vi "Delete Ansiotropic Filter 32f.vi"(8 "Error In":errorcluster, 11 "Anisotropic Filter Object":T1={"Device In"=0, "Convolution Object"={"Device In"=0, "Program Handle"=0, "Kernel Memory Object"={"Device ID"=0, "Memeroy ID"=0, "Dimension"={"Depth"=0, "Height"=0, "Width"=0}, "Memory Type"=enum."32f"}, "Convolved Memory Object"={"Device ID"=0, "Memeroy ID"=0, "Dimension"={"Depth"=0, "Height"=0, "Width"=0}, "Memory Type"=enum."32f"}}, "Imag Kernel"=[], "Real Kernel"=[], "Convolved Buffer"={"Device ID"=0, "Memeroy ID"=0, "Dimension"={"Depth"=0, "Height"=0, "Width"=0}, "Memory Type"=enum."32f"}, "Program Handle"=0, "Ansiotropic Filter Parameters"={"Time Step"=0.0, "Total Time"=0.5, "Std. Deviation"=0.0, "Gaussian Filter X Size"=1, "Gaussian Filter Y Size"=1, "Gaussian Filter Z Size"=1}, "Raw Data"={"Device ID"=0, "Memeroy ID"=0, "Dimension"={"Depth"=0, "Height"=0, "Width"=0}, "Memory Type"=enum."32f"}, "Buffer 3"={"Device ID"=0, "Memeroy ID"=0, "Dimension"={"Depth"=0, "Height"=0, "Width"=0}, "Memory Type"=enum."32f"}, "Dimensions"={"Depth"=1, "Height"=1, "Width"=1}} {"Dimensions"."Width" min=1; "Dimensions"."Height" min=1; "Dimensions"."Depth" min=1; "Buffer 3"."Dimension"."Width" min=1; "Buffer 3"."Dimension"."Height" min=1; "Buffer 3"."Dimension"."Depth" min=1; "Raw Data"."Dimension"."Width" min=1; "Raw Data"."Dimension"."Height" min=1; "Raw Data"."Dimension"."Depth" min=1; "Ansiotropic Filter Parameters"."Gaussian Filter Z Size" min=1 max=99 step=2; "Ansiotropic Filter Parameters"."Gaussian Filter Y Size" min=1 max=99 step=2; "Ansiotropic Filter Parameters"."Gaussian Filter X Size" min=1 max=99 step=2; "Convolved Buffer"."Dimension"."Width" min=1; "Convolved Buffer"."Dimension"."Height" min=1; "Convolved Buffer"."Dimension"."Depth" min=1; "Convolution Object"."Convolved Memory Object"."Dimension"."Width" min=1; "Convolution Object"."Convolved Memory Object"."Dimension"."Height" min=1; "Convolution Object"."Convolved Memory Object"."Dimension"."Depth" min=1; "Convolution Object"."Kernel Memory Object"."Dimension"."Width" min=1; "Convolution Object"."Kernel Memory Object"."Dimension"."Height" min=1; "Convolution Object"."Kernel Memory Object"."Dimension"."Depth" min=1}) -> (0 "Error Out":errorcluster)   [LabVIEW 2012, in "OpenCLV x64.lvlib"]
doc: "Deletes the program and memory objects associated with an Anisotropic Filter Object."
uses:
  OpenCLV x64.lvlib
  Controls/Anisotropic Filter Object.ctl
  Controls/Device ID.ctl
  Controls/Convolution Object.ctl
  Controls/Program Handle.ctl
  Controls/Memory Object.ctl
  Controls/Memory ID.ctl
  User Controls/Array Dimensions.ctl
  Controls/Memory Type.ctl
  Controls/Anisotropic Filter Parameters.ctl
  Convolution/Delete Convolution 32f.vi
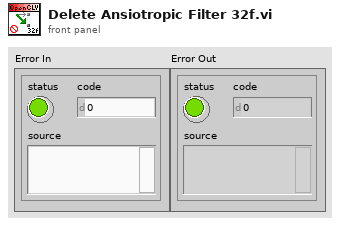
[diagram p1: front panel]
types:
  T1 = typedef "OpenCLV x64.lvlib/Anisotropic Filter Object.ctl" = cluster{"Device In":T2, "Convolution Object":T3, "Imag Kernel":sgl[][][], "Real Kernel":sgl[][][], "Convolved Buffer":T5, "Program Handle":T4, "Ansiotropic Filter Parameters":T9, "Raw Data":T5, "Buffer 3":T5, "Dimensions":T7}
  T2 = typedef "OpenCLV x64.lvlib/Device ID.ctl" = u64
  T3 = typedef "OpenCLV x64.lvlib/Convolution Object.ctl" = cluster{"Device In":T2, "Program Handle":T4, "Kernel Memory Object":T5, "Convolved Memory Object":T5}
  T4 = typedef "OpenCLV x64.lvlib/Program Handle.ctl" = u64
  T5 = typedef "OpenCLV x64.lvlib/Memory Object.ctl" = cluster{"Device ID":T2, "Memeroy ID":T6, "Dimension":T7, "Memory Type":T8}
  T6 = typedef "OpenCLV x64.lvlib/Memory ID.ctl" = u64
  T7 = typedef "Array Dimensions.ctl" = cluster{"Depth":u64, "Height":u64, "Width":u64}
  T8 = typedef "OpenCLV x64.lvlib/Memory Type.ctl" = enum16{"32f", "u8", "i8", "u16", "i16", "u32", "i32", "64f"}
  T9 = typedef "OpenCLV x64.lvlib/Anisotropic Filter Parameters.ctl" = cluster{"Time Step":sgl, "Total Time":sgl, "Std. Deviation":sgl, "Gaussian Filter X Size":u32, "Gaussian Filter Y Size":u32, "Gaussian Filter Z Size":u32}
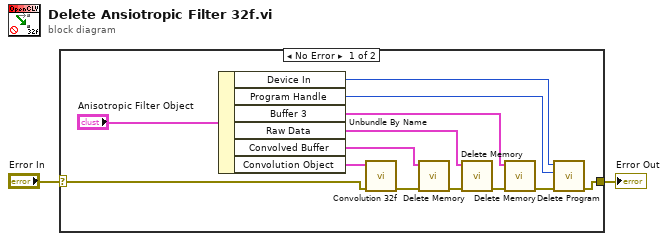
[diagram p0: block diagram]
diagram:
  n1 = case shown="No Error" "Error In" {
    selector: "Error In" -> [w3 w16]
    tunnel: [w8 w16] -> w1
    frame No Error {
      n2 = Unbundle By Name("Anisotropic Filter Object") -> ("Device In"=w7:T2, "Program Handle"=w9:T4, "Buffer 3"=w11:T5, "Raw Data"=w13:T5, "Convolved Buffer"=w4:T5, "Convolution Object"=w14:T3)
      n3 = call-poly "Convolution 32f.vi"("Error In"=w3, "Convolution Object"=w14) -> ("Error Out"=w6:errorcluster)  [unwired: 9 in]
      n4 = call "Delete Memory.vi"("Error In"=w6, "Memory Object In"=w4) -> ("Error Out"=w5:errorcluster)  [unwired: 8 in, 1 out]
      n5 = call "Delete Memory.vi"("Error In"=w5, "Memory Object In"=w13) -> ("Error Out"=w12:errorcluster)  [unwired: 8 in, 1 out]
      n6 = call "Delete Memory.vi"("Error In"=w12, "Memory Object In"=w11) -> ("Error Out"=w10:errorcluster)  [unwired: 8 in, 1 out]
      n7 = call "Delete Program.vi"("Error In"=w10, "Program In"=w9, "Device ID"=w7) -> ("Error Out"=w8:errorcluster)  [unwired: 8 in]
    }
    frame Error {
    }
  }
  "Error Out" <- w1
